vi "Val Change Checker.vi"(1 "Current Value in":variant) -> (0 "Value Change?":bool)   [LabVIEW 2018]
doc: "Outputs true when the input changes value or if it is the First Call."
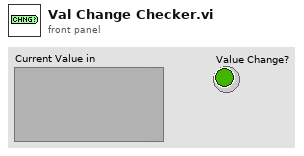
[diagram p1: front panel]
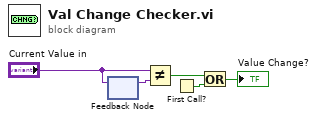
[diagram p0: block diagram]
diagram:
  n1 = feedback #1() -> (w1:variant)  [unwired: 1 in]
  n2 = feedback-in #1("Current Value in") -> ()
  n3 = Not Equal?(x="Current Value in", y=w1) -> (x != y?=w3:bool)
  n4 = First Call?() -> (First Call?: T/F=w4:bool)
  n5 = Or(x=w3, y=w4) -> (x .or. y?=→"Value Change?":bool)
